vi "Translate Data to Virtual Device Data.vi"(10 "PV Data":T1) -> (1 "Data Array":u16[](array[numeric]), 2 "Address":u16)   [LabVIEW 2015, in "AE75TX Actor.lvlib" / "AE75TX.lvclass"]
doc: "This code converts the data coming from the real device to the format the EMS understands."
uses:
  AE75TX.lvclass
  Controls/PV Full Data Cluster.ctl
  Controls/PV Standard Value Cluster.ctl
  Utilities/Modbus Data Conversion.llb/Modbus Data Conversion.lvlib
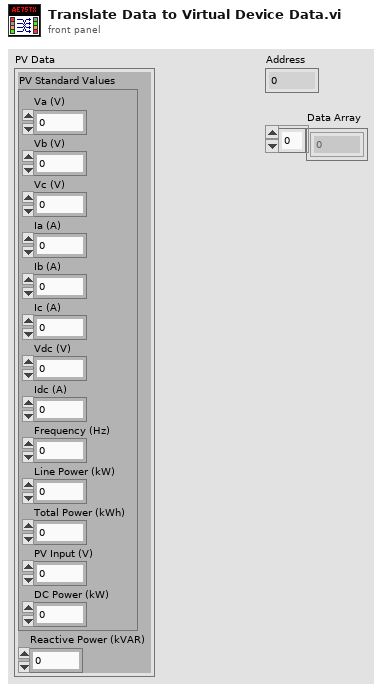
[diagram p1: front panel]
types:
  T1 = typedef "AE75TX Actor.lvlib/AE75TX.lvclass/PV Full Data Cluster.ctl" = cluster{"PV Standard Values":T2, "Reactive Power (kVAR)":sgl}
  T2 = typedef "AE75TX Actor.lvlib/AE75TX.lvclass/PV Standard Value Cluster.ctl" = cluster{"Va (V)":sgl, "Vb (V)":sgl, "Vc (V)":sgl, "Ia (A)":sgl, "Ib (A)":sgl, "Ic (A)":sgl, "Vdc (V)":sgl, "Idc (A)":sgl, "Frequency (Hz)":sgl, "Line Power (kW)":sgl, "Total Power (kWh)":u32, "PV Input (V)":sgl, "DC Power (kW)":sgl}
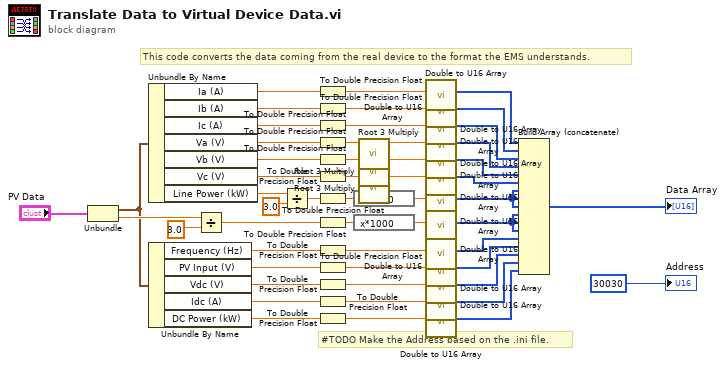
[diagram p0: block diagram]
diagram:
  # "This code converts the data coming from the real device to the format the EMS understands."
  # "#TODO Make the Address based on the .ini file."
  n1 = Unbundle("PV Data") -> ("PV Standard Values"=w23:T2, "Reactive Power (kVAR)"=w49:sgl)
  n2 = Unbundle By Name(w23) -> ("Ia (A)"=w25:sgl, "Ib (A)"=w26:sgl, "Ic (A)"=w27:sgl, "Va (V)"=w28:sgl, "Vb (V)"=w29:sgl, "Vc (V)"=w30:sgl, "Line Power (kW)"=w24:sgl)
  n3 = Unbundle By Name(w23) -> ("Frequency (Hz)"=w47:sgl, "PV Input (V)"=w46:sgl, "Vdc (V)"=w45:sgl, "Idc (A)"=w39:sgl, "DC Power (kW)"=w38:sgl)
  n4 = Divide(x=w49, y=sgl 3.0) -> (x/y=w37:sgl)
  n5 = Divide(x=w24, y=sgl 3.0) -> (x/y=w36:sgl)
  n6 = To Double Precision Float(number=w25) -> (double precision float=w31:dbl)
  n7 = To Double Precision Float(number=w26) -> (double precision float=w32:dbl)
  n8 = To Double Precision Float(number=w27) -> (double precision float=w33:dbl)
  n9 = To Double Precision Float(number=w28) -> (double precision float=w9:dbl)
  n10 = To Double Precision Float(number=w29) -> (double precision float=w4:dbl)
  n11 = To Double Precision Float(number=w30) -> (double precision float=w5:dbl)
  n12 = To Double Precision Float(number=w36) -> (double precision float=w34:dbl)
  n13 = To Double Precision Float(number=w37) -> (double precision float=w2:dbl)
  n14 = To Double Precision Float(number=w47) -> (double precision float=w44:dbl)
  n15 = To Double Precision Float(number=w46) -> (double precision float=w43:dbl)
  n16 = To Double Precision Float(number=w45) -> (double precision float=w42:dbl)
  n17 = To Double Precision Float(number=w39) -> (double precision float=w41:dbl)
  n18 = To Double Precision Float(number=w38) -> (double precision float=w40:dbl)
  n19 = expression code="x*1000"(w34) -> (w3:dbl)
  n20 = expression code="x*1000"(w2) -> (w1:dbl)
  n21 = call "Root 3 Multiply.vi"("RMS Line to Neutral"=w9) -> ("RMS Line to Line"=w8:dbl)  [unwired: 10 in]
  n22 = call "Root 3 Multiply.vi"("RMS Line to Neutral"=w4) -> ("RMS Line to Line"=w7:dbl)  [unwired: 10 in]
  n23 = call "Root 3 Multiply.vi"("RMS Line to Neutral"=w5) -> ("RMS Line to Line"=w6:dbl)  [unwired: 10 in]
  n24 = call "Double to U16 Array.vi"("Double"=w31) -> ("U16 Array"=w22:u16[])  [unwired: 10 in]
  n25 = call "Double to U16 Array.vi"("Double"=w32) -> ("U16 Array"=w21:u16[])  [unwired: 10 in]
  n26 = call "Double to U16 Array.vi"("Double"=w33) -> ("U16 Array"=w20:u16[])  [unwired: 10 in]
  n27 = call "Double to U16 Array.vi"("Double"=w8) -> ("U16 Array"=w19:u16[])  [unwired: 10 in]
  n28 = call "Double to U16 Array.vi"("Double"=w7) -> ("U16 Array"=w18:u16[])  [unwired: 10 in]
  n29 = call "Double to U16 Array.vi"("Double"=w6) -> ("U16 Array"=w17:u16[])  [unwired: 10 in]
  n30 = call "Double to U16 Array.vi"("Double"=w3) -> ("U16 Array"=w16:u16[])  [unwired: 10 in]
  n31 = call "Double to U16 Array.vi"("Double"=w1) -> ("U16 Array"=w15:u16[])  [unwired: 10 in]
  n32 = call "Double to U16 Array.vi"("Double"=w44) -> ("U16 Array"=w14:u16[])  [unwired: 10 in]
  n33 = call "Double to U16 Array.vi"("Double"=w43) -> ("U16 Array"=w13:u16[])  [unwired: 10 in]
  n34 = call "Double to U16 Array.vi"("Double"=w42) -> ("U16 Array"=w12:u16[])  [unwired: 10 in]
  n35 = call "Double to U16 Array.vi"("Double"=w41) -> ("U16 Array"=w11:u16[])  [unwired: 10 in]
  n36 = call "Double to U16 Array.vi"("Double"=w40) -> ("U16 Array"=w10:u16[])  [unwired: 10 in]
  n37 = Build Array (concatenate)(w22, w21, w20, w19, w18, w17, w16, w16, w16, w15, w15, w15, w14, w13, w12, w11, w10) -> (→"Data Array":u16[])
  "Address" <- u16 30030 ("Address")
